vi "Type Color.vi"(11 "IntegerPanel in":refnum<class "IntegerPanel.lvclass">) -> (2 "Type Color":u32(colorbox))   [LabVIEW 2020, in "Conditum-Tools.lvlib" / "IntegerPanel.lvclass"]
uses:
  IntegerPanel.lvclass
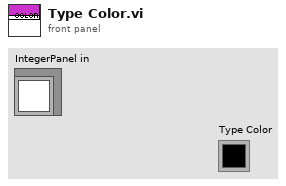
[diagram p1: front panel]
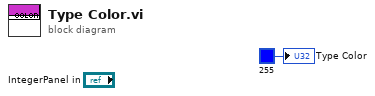
[diagram p0: block diagram]
diagram:
  "Type Color" <- u32 255 ("Type Color")
